vi "XYMovFormTest.vi"() -> ()   [LabVIEW 2013]
uses:
  <vilib>/Instr/_visa.llb/VISA Configure Serial Port (Instr).vi
panel:
  out "read buffer 2":string
  in  "milliseconds to wait":u32
  in  "stop":bool
  out "read buffer":string
  in  "Path":path
  in  "XYZ":refnum<visa-resource-name>
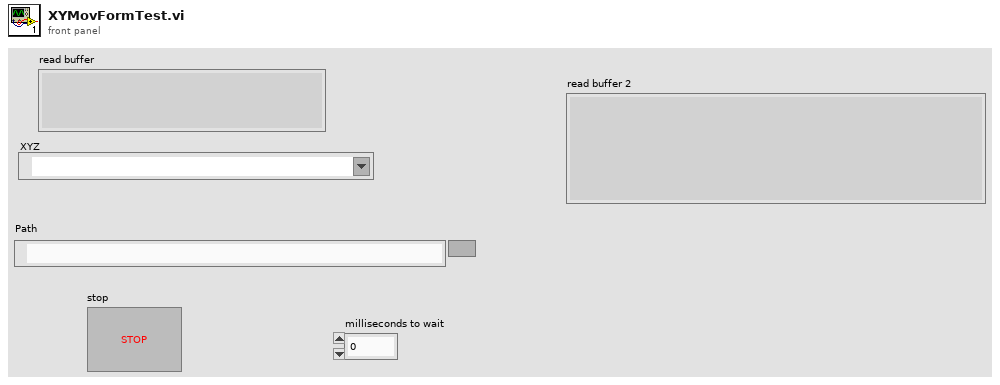
[diagram p1: front panel]
types:
  T1 = enum16{"open", "replace", "create", "open or create", "replace or create", "replace or create with confirmation"}
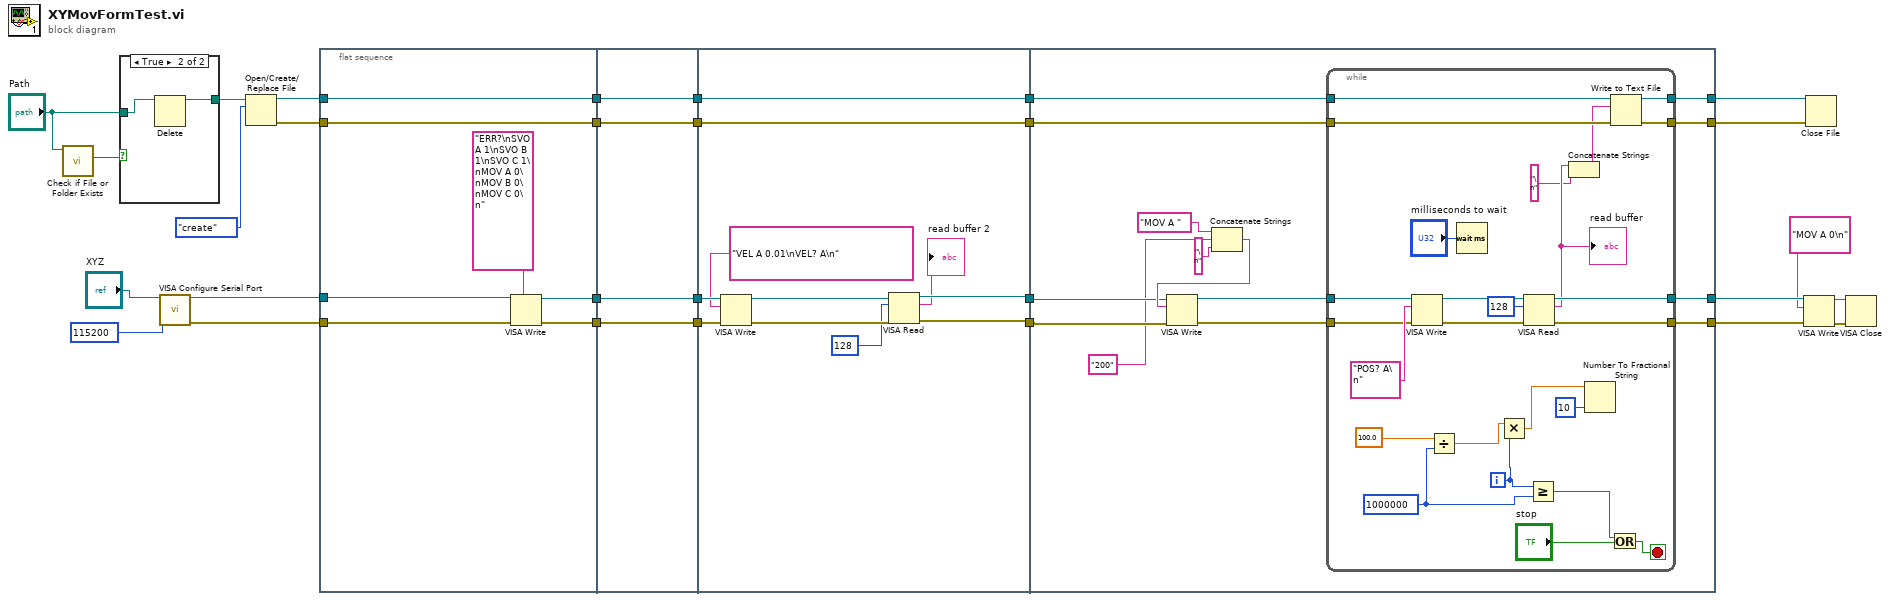
[diagram p0: block diagram]
diagram:
  n1 = call <vilib>:"Check if File or Folder Exists.vi"("path"="Path") -> ("file or folder exists?"=w25:bool)  [unwired: 8 in, 2 out]
  n2 = case shown="True" w25 {
    tunnel: "Path" -> [w30 w32]
    tunnel: [w30 w31] -> w22
    frame False {
    }
    frame True {
      n3 = Delete(path (use dialog)=w32) -> (deleted path=w31:path)  [unwired: 4 in, 2 out]
    }
  }
  n4 = call-poly "VISA Configure Serial Port"("VISA resource name"="XYZ", "baud rate (9600)"=u32 115200) -> ("VISA resource name out"=w27:refnum<visa-resource-name>, "error out"=w26:errorcluster)  [unwired: 12 in]
  n5 = Open/Create/Replace File(file path (use dialog)=w22, operation (0:open)=T1."create") -> (refnum out=w21:refnum<file>, error out=w20:errorcluster)  [unwired: 4 in, 1 out]
  n6 = flat-sequence {
    tunnel: w27 -> [w39]
    tunnel: w26 -> [w38]
    tunnel: [w36] -> w19
    tunnel: [w35] -> w18
    tunnel: w21 -> [w34]
    tunnel: w20 -> [w33]
    tunnel: [w34] -> w17
    tunnel: [w33] -> w16
    tunnel: w19 -> [w43]
    tunnel: [w43] -> w8
    tunnel: w18 -> [w42]
    tunnel: [w42] -> w6
    tunnel: w17 -> [w41]
    tunnel: [w41] -> w4
    tunnel: w16 -> [w40]
    tunnel: [w40] -> w2
    tunnel: w8 -> [w52]
    tunnel: [w47] -> w7
    tunnel: w6 -> [w51]
    tunnel: [w46] -> w5
    tunnel: w4 -> [w54]
    tunnel: [w54] -> w3
    tunnel: w2 -> [w53]
    tunnel: [w53] -> w1
    tunnel: w7 -> [w59]
    tunnel: w5 -> [w58]
    tunnel: w3 -> [w68]
    tunnel: w1 -> [w67]
    tunnel: [w66] -> w15
    tunnel: [w65] -> w14
    tunnel: [w64] -> w13
    tunnel: [w63] -> w12
    frame #0 {
      n7 = VISA Write(VISA resource name=w39, write buffer="ERR?\nSVO A 1\nSVO B 1\nSVO C 1\nMOV A 0\nMOV B 0\nMOV C 0\n", error in (no error)=w38) -> (VISA resource name out=w36:refnum<visa-resource-name>, error out=w35:errorcluster)  [unwired: 1 out]
    }
    frame #1 {
    }
    frame #2 {
      n8 = VISA Write(VISA resource name=w52, write buffer="VEL A 0.01\nVEL? A\n", error in (no error)=w51) -> (VISA resource name out=w49:refnum<visa-resource-name>, error out=w48:errorcluster)  [unwired: 1 out]
      n9 = VISA Read(VISA resource name=w49, byte count=u32 128, error in (no error)=w48) -> (VISA resource name out=w47:refnum<visa-resource-name>, read buffer=→"read buffer 2":string, error out=w46:errorcluster)  [unwired: 1 out]
    }
    frame #3 {
      n10 = Concatenate Strings("MOV A " ("write buffer"), "200", "\n" ("string")) -> (w61:string)
      n11 = VISA Write(VISA resource name=w59, write buffer=w61, error in (no error)=w58) -> (VISA resource name out=w57:refnum<visa-resource-name>, error out=w56:errorcluster)  [unwired: 1 out]
      n12 = while {
        tunnel: w68 -> [w87]
        tunnel: w67 -> [w86]
        tunnel: [w91] -> w64
        tunnel: [w90] -> w63
        tunnel: [w85] -> w66
        tunnel: [w84] -> w65
        tunnel: w57 -> [w70]
        tunnel: w56 -> [w69]
        i -> [w74]
        stop <- w80 stop-if-true
        w77 = 1000000 ("y")
        n13 = VISA Write(VISA resource name=w70, write buffer="POS? A\n", error in (no error)=w69) -> (VISA resource name out=w93:refnum<visa-resource-name>, error out=w92:errorcluster)  [unwired: 1 out]
        n14 = Divide(x=100.0, y=w77) -> (x/y=w75:dbl)
        n15 = Wait (ms)(milliseconds to wait="milliseconds to wait") -> ()  [unwired: 1 out]
        n16 = Multiply(x=w75, y=w74) -> (x*y=w72:dbl)
        n17 = VISA Read(VISA resource name=w93, byte count=u32 128, error in (no error)=w92) -> (VISA resource name out=w91:refnum<visa-resource-name>, read buffer=w83:string, error out=w90:errorcluster)  [unwired: 1 out]
        "read buffer" <- w83
        n18 = Greater Or Equal?(x=w74, y=w77) -> (x >= y?=w78:bool)
        n19 = Concatenate Strings(w83, "\n" ("string")) -> (w81:string)
        n20 = Number To Fractional String(number=w72, precision (6)=i16 10) -> ()  [unwired: 2 in, 1 out]
        n21 = Or(x=w78, y="stop") -> (x .or. y?=w80:bool)
        n22 = Write to Text File(file (use dialog)=w87, text=w81, error in=w86) -> (refnum out=w85:refnum<file>, error out=w84:errorcluster)  [unwired: 1 in, 1 out]
      }
    }
  }
  n23 = VISA Write(VISA resource name=w13, write buffer="MOV A 0\n", error in (no error)=w12) -> (VISA resource name out=w11:refnum<visa-resource-name>, error out=w10:errorcluster)  [unwired: 1 out]
  n24 = Close File(refnum=w15, error in=w14) -> ()  [unwired: 2 out]
  n25 = VISA Close(VISA resource name=w11, error in (no error)=w10) -> ()  [unwired: 1 out]
